vi "zlgcan_demo_CANET.vi"() -> ()   [LabVIEW 2018]
uses:
  data_type/ZCAN_InitCAN_setting_CANET.ctl
panel:
  in  "本地端口":u32=6001
  in  "TCP模式":u32(ring) items=["客户端（client）", "服务器（server）"]
  in  "工作端口":u32=4001
  in  "IP":string="192.168.0.178"
  in  "设备索引":u32(ring) items=["0", "1", "2", "3"]
  in  "设备类型":u32(ring)=17 items=["CANET-UDP"=12, "CANET-TCP"=17, "USBCAN-II"=4, "USBCAN-E-U"=20, "USBCANFD-100U"=42, "USBCANFD-200U"=41, "PCIE-CANFD-100U"=38, "PCIE-CANFD-200U"=39, "PCIE-CANFD-400U"=40, "云设备"=46]
  in  "开启CAN":bool
  in  "stop":bool
  out "can_index_handle(out)":u32
  out "Device_handle(out)":u32
  in  "ID":u32 format="0x%08x"
  in  "数据长度(最大8字节)":u8=8 max=8
  in  "Data Byte 8":u8 caption="data88" format="%.0x"
  in  "Data Byte 7":u8 caption="data7" format="%.0x"
  in  "Data Byte 6":u8 caption="data6" format="%.0x"
  in  "Data Byte 5":u8 caption="data5" format="%.0x"
  in  "Data Byte 4":u8 caption="data4" format="%.0x"
  in  "Data Byte 3":u8 caption="data3" format="%.0x"
  in  "Data Byte 2":u8 caption="data2" format="%.0x"
  in  "Data Byte 1":u8 caption="data1" format="%.0x"
  in  "帧格式":u32(ring) items=["数据帧", "远程帧"]
  in  "发送方式":u32(ring) items=["正常发送", "单次发送", "自发自收", "单次自发自收"]
  in  "帧类型":u32(ring) items=["标准帧", "扩展帧"]
  in  "每次发送帧数":u32=1
  in  "发送":bool
  in  "ZCAN_InitCAN_setting_CANET":T1
  out "已接收帧数":u32
  out "String":string
  # "停止程序前，需要先关闭CAN卡"
  # "当CANET的工作模式为：\n\n1. 客户端（TCP Client）\n\n   LabVIEW 设备型号选择【 CANET-TCP】\n\n   TCP模式选择【服务器 TCP Sever】\n\n   填写电脑本机IP+本地端口。\n\n2. 服务器（TCP Sever）\n\n   LabVIEW 设备型号选择【 CANET-TCP】\n\n   TCP模式选择【客户端 TCP Client】\n\n   填写CANET的 IP +工作端口\n\n3. UDP\n\n   LabVIEW 设备型号选择【 CANET-UDP】\n\n   填写CANET的IP+工作端口+本地端口"
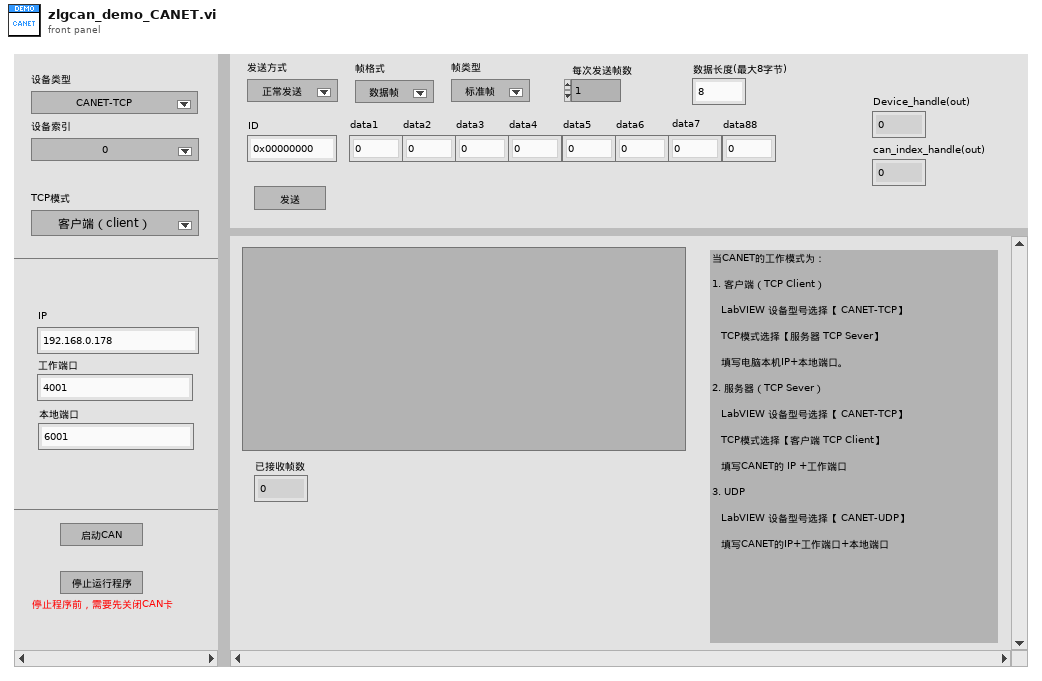
[diagram p1: front panel]
types:
  T1 = typedef "ZCAN_InitCAN_setting_CANET.ctl" = cluster{"tcp_type":u32, "work_port":u32, "local_port":u32, "IP":string}
  T2 = cluster{"[0]":u8, "[1]":u8, "[2]":u8, "[3]":u8, "[4]":u8, "[5]":u8, "[6]":u8, "[7]":u8}
  T3 = cluster{u32, u8, u8, u8, u8, cluster{"[0]":u8, "[1]":u8, "[2]":u8, "[3]":u8, "[4]":u8, "[5]":u8, "[6]":u8, "[7]":u8}, u64}[]
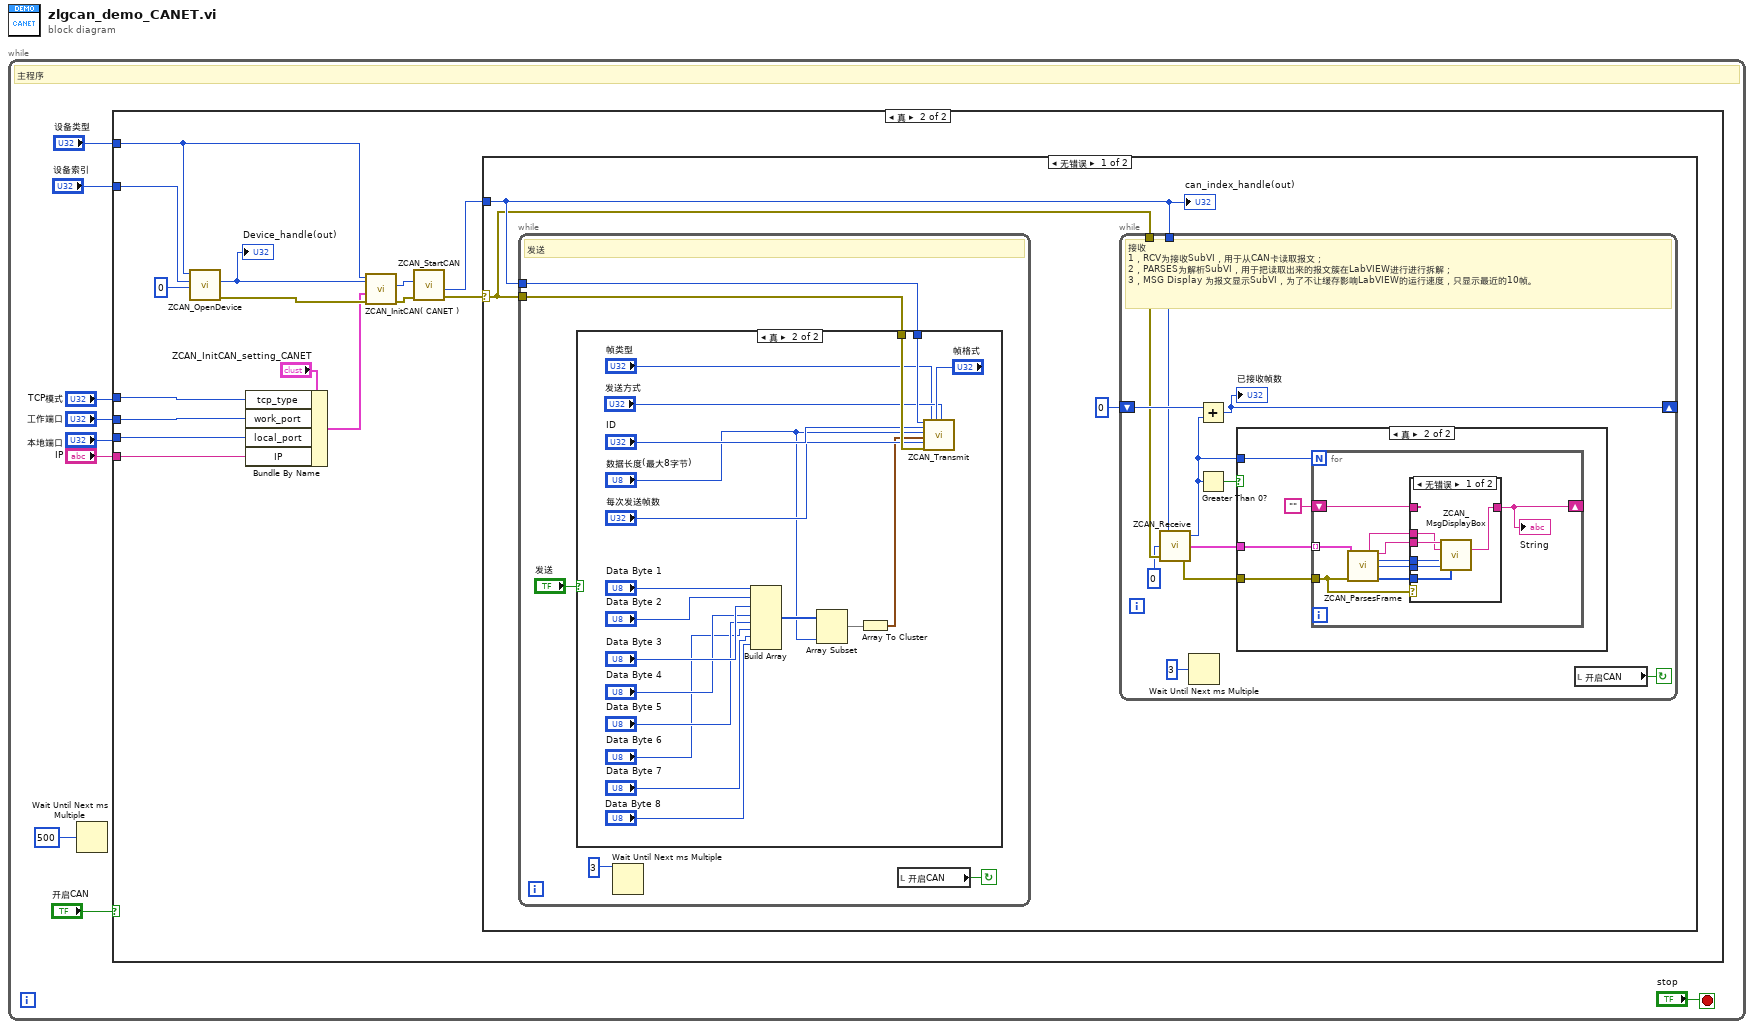
[diagram p0: block diagram]
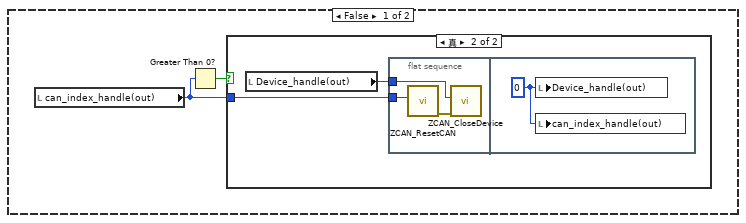
[diagram p2: hidden frame]
diagram:
  n1 = while {
    stop <- "stop" stop-if-true
    # "主程序"
    n2 = Wait Until Next ms Multiple(millisecond multiple=u32 500) -> ()  [unwired: 1 out]
    n3 = case shown="真" "开启CAN" {
      tunnel: "设备类型" -> [_ w19]
      tunnel: "设备索引" -> [_ w30]
      tunnel: "IP" -> [_ w23]
      tunnel: "TCP模式" -> [_ w24]
      tunnel: "工作端口" -> [_ w22]
      tunnel: "本地端口" -> [_ w21]
      frame False {
        n4 = local read "can_index_handle(out)"() -> (w10:u32)
        n5 = Greater Than 0?(x=w10) -> (x > 0?=w11:bool)
        n6 = case shown="真" w11 {
          tunnel: w10 -> [_ w13]
          frame False {
          }
          frame True {
            n7 = local read "Device_handle(out)"() -> (w12:u32)
            n8 = flat-sequence {
              tunnel: w13 -> [w15]
              tunnel: w12 -> [w14]
              frame #0 {
                n9 = call "ZCAN_ResetCAN.vi"("can_handle"=w15) -> ("error out"=w16:errorcluster)  [unwired: 9 in, 1 out]
                n10 = call "ZCAN_CloseDevice.vi"("error in (no error)"=w16, "device_handle"=w14) -> ()  [unwired: 8 in, 2 out]
              }
              frame #1 {
                w17 = u32 0 ("can_index_handle(out)")
                n11 = local write "Device_handle(out)"(w17) -> ()
                n12 = local write "can_index_handle(out)"(w17) -> ()
              }
            }
          }
        }
      }
      frame True {
        n13 = call "ZCAN_OpenDevice.vi"("reserved"=0, "device_index"=w30, "device_type"=w19) -> ("error out"=w28:errorcluster, "DEVICE_HANDLE"=w18:u32)  [unwired: 7 in]
        "Device_handle(out)" <- w18
        n14 = Bundle By Name(cluster="ZCAN_InitCAN_setting_CANET", "tcp_type"=w24, "work_port"=w22, "local_port"=w21, "IP"=w23) -> (w20:T1)
        n15 = call "ZCAN_InitCAN( CANET ).vi"("error in (no error)"=w28, "ZCAN_InitCAN_setting_CANET"=w20, "device_hande"=w18, "设备类型"=w19) -> ("error out"=w27:errorcluster, "can_index_handle"=w26:u32)  [unwired: 2 in]
        n16 = call "ZCAN_StartCAN.vi"("error in (no error)"=w27, "can_index_handle"=w26) -> ("error out"=w32:errorcluster, "can_index_handle(out)"=w31:u32)  [unwired: 7 in, 1 out]
        n17 = case shown="无错误" w32 {
          selector: w32 -> [w34 _]
          tunnel: w31 -> [w35 _]
          frame No Error {
            n18 = while {
              tunnel: w35 -> [w69]
              tunnel: w34 -> [w67]
              stop <- w68 continue-if-true
              # "发送"
              n19 = case shown="真" "发送" {
                tunnel: w69 -> [_ w90]
                tunnel: w67 -> [_ w89]
                frame False {
                }
                frame True {
                  n20 = Build Array("Data Byte 1", "Data Byte 2", "Data Byte 3", "Data Byte 4", "Data Byte 5", "Data Byte 6", "Data Byte 7", "Data Byte 8") -> (w76:u8[])
                  n21 = Array Subset(array=w76, length="数据长度(最大8字节)") -> (w74:u8[])  [unwired: 1 in]
                  n22 = Array To Cluster(array=w74) -> (cluster=w73:T2)
                  n23 = call "ZCAN_Transmit.vi"("can_index_handle"=w90, "ID"="ID", "数据长度"="数据长度(最大8字节)", "DATA"=w73, "每次发送帧数"="每次发送帧数", "error in (no error)"=w89, "帧类型"="帧类型", "帧格式"="帧格式", "发送方式"="发送方式") -> ()  [unwired: 10 in, 1 out]
                }
              }
              n24 = Wait Until Next ms Multiple(millisecond multiple=u32 3) -> ()  [unwired: 1 out]
              n25 = local read "开启CAN"() -> (w68:bool)
            }
            n26 = while {
              tunnel: w34 -> [w43]
              tunnel: w35 -> [w41]
              shift-right: [w44] -> _
              shift-left: 0 -> [w45]
              stop <- w36 continue-if-true
              # "接收\n1，RCV为接收SubVI，用于从CAN卡读取报文；\n2，PARSES为解析SubVI，用于把读取出来的报文簇在LabVIEW进行进行拆解；\n3，MSG Display 为报文显示SubVI，为了不让缓存影响LabVIEW的运行速度，只显示最近的10帧。"
              n27 = call "ZCAN_Receive.vi"("error in (no error)"=w43, "type"=u8 0, "can_handle"=w41) -> ("error out"=w39:errorcluster, "Receive"=w40:T3, "Receive_Num"=w38:u32)
              n28 = Wait Until Next ms Multiple(millisecond multiple=u32 3) -> ()  [unwired: 1 out]
              n29 = Add(x=w45, y=w38) -> (x+y=w44:u32)
              "已接收帧数" <- w44
              n30 = Greater Than 0?(x=w38) -> (x > 0?=w37:bool)
              n31 = case shown="真" w37 {
                tunnel: w38 -> [_ w50]
                tunnel: w40 -> [_ w49]
                tunnel: w39 -> [_ w48]
                frame False {
                }
                frame True {
                  n32 = for {
                    N: w50 -> [_]
                    tunnel: w49 -> [w57] mode=indexing
                    tunnel: w48 -> [w56]
                    shift-right: [w59] -> _
                    shift-left: "" -> [w58]
                    n33 = call "ZCAN_ParsesFrame.vi"("ZCAN_Receive_Data"=w57, "error in (no error)"=w56) -> ("帧格式"=w51:string, "帧类型"=w52:string, "ID"=w53:u32, "data_len"=w55:u8, "data"=w54:u8[])  [unwired: 8 in, 1 out]
                    n34 = case shown="无错误" w56 {
                      tunnel: [w65 w66] -> w59
                      tunnel: w58 -> [_ w66]
                      tunnel: w55 -> [w64 _]
                      tunnel: w54 -> [w63 _]
                      tunnel: w53 -> [w62 _]
                      tunnel: w52 -> [w61 _]
                      tunnel: w51 -> [w60 _]
                      frame No Error {
                        n35 = call "ZCAN_MsgDisplayBox.vi"("帧类型"=w61, "ID"=w62, "帧格式"=w60, "Message Data"=w63, "data_len"=w64) -> ("Output String"=w65:string)  [unwired: 10 in]
                      }
                      frame Error {
                      }
                    }
                    "String" <- w59
                  }
                }
              }
              n36 = local read "开启CAN"() -> (w36:bool)
            }
            "can_index_handle(out)" <- w35
          }
          frame Error {
          }
        }
      }
    }
  }
